vi "Read Global Acceleration.vi"(8 "error in (no error)":errorcluster, 11 "PhysicsSystem in":refnum<class "PhysicsSystem.lvclass">) -> (0 "error out":errorcluster, 2 "Vector2.lvclass":refnum<class "Vector2.lvclass">, 3 "PhysicsSystem out":refnum<class "PhysicsSystem.lvclass">)   [LabVIEW 2022 SP3, in "PhysicsSystem.lvclass"]
uses:
  PhysicsSystem.lvclass
  PhysicsSystem.lvclass/PhysicsSystem.ctl
  Math/Vector2/Vector2.lvclass
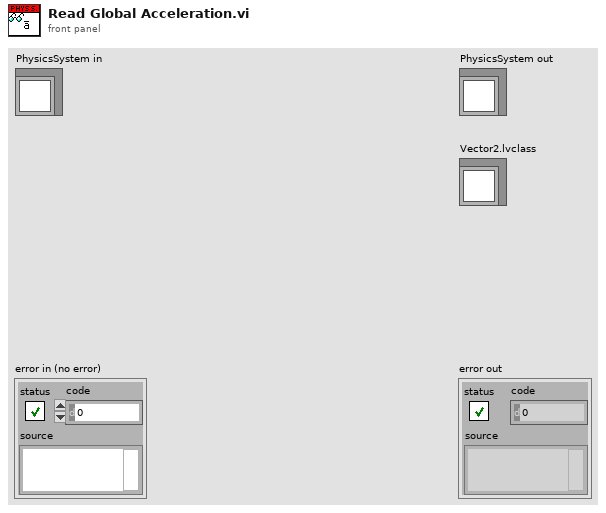
[diagram p1: front panel]
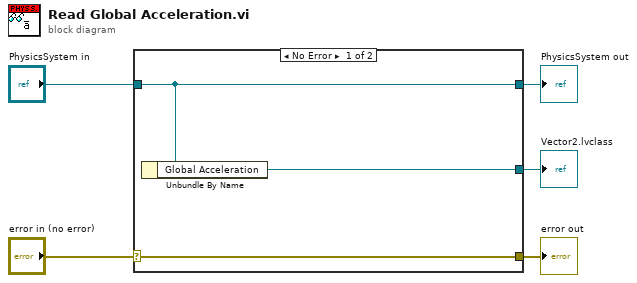
[diagram p0: block diagram]
diagram:
  n1 = case shown="No Error" "error in (no error)" {
    selector: "error in (no error)" -> [w8 w9]
    tunnel: [w8 w9] -> w4
    tunnel: [w7 w10] -> w2
    tunnel: "PhysicsSystem in" -> [w7 w10]
    tunnel: [w6 _] -> w1
    frame No Error {
      n2 = Unbundle By Name(w7) -> ("Global Acceleration"=w6:refnum<class "Vector2.lvclass">)
    }
    frame Error {
    }
  }
  "error out" <- w4
  "PhysicsSystem out" <- w2
  "Vector2.lvclass" <- w1
